vi "GetState.vi"(6 "error in (no error)":errorcluster, 8 "IMU Channel":tag="A/I2C", 9 "LIDAR Channel":tag="B/I2C") -> (0 "error out":errorcluster, 1 "Height":dbl, 2 "Angular Velocity":dbl[](array[numeric]), 3 "Acceleration":dbl[](array[numeric]))   [LabVIEW 2017]
panel:
  in  "Acceleration Factor (experimentally determined)":dbl format="%#_13g"
  out "MyRIO Acceleration":dbl[](array[numeric])
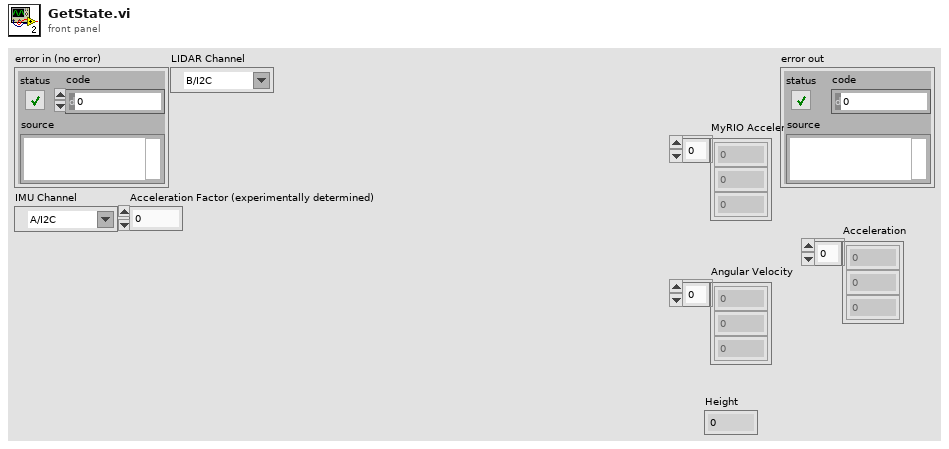
[diagram p1: front panel]
types:
  T1 = cluster{"X-axis":i16, "Y-axis":i16, "Z-axis":i16}
  T2 = cluster{"X-Axis":dbl, "Y-Axis":dbl, "Z-Axis":dbl}
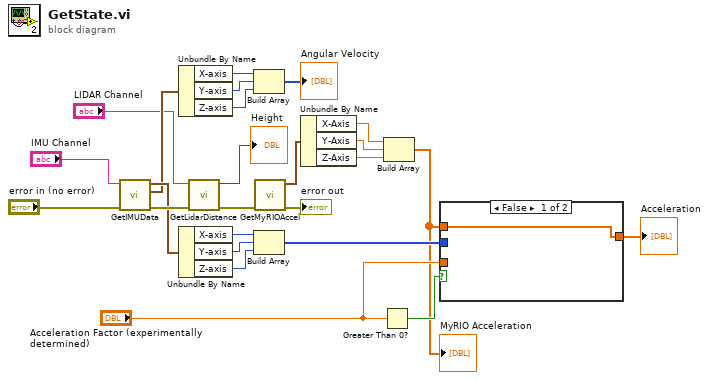
[diagram p0: block diagram]
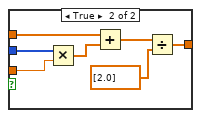
[diagram p2: hidden frame]
diagram:
  n1 = call "GetIMUData.vi"("error in (no error)"="error in (no error)", "Channel Name"="IMU Channel") -> ("error out"=w23:errorcluster, "GyroData"=w18:T1, "AccelData"=w19:T1)  [unwired: 7 in]
  n2 = Unbundle By Name(w18) -> ("X-axis"=w12:i16, "Y-axis"=w11:i16, "Z-axis"=w10:i16)
  n3 = Unbundle By Name(w19) -> ("X-axis"=w8:i16, "Y-axis"=w7:i16, "Z-axis"=w6:i16)
  n4 = call "GetLidarDistance.vi"("error in"=w23, "Channel Name"="LIDAR Channel") -> ("error out"=w22:errorcluster, "(hi.lo)"=→"Height":u16)  [unwired: 8 in]
  n5 = Build Array(w12, w11, w10) -> (→"Angular Velocity":i16[])
  n6 = Build Array(w8, w7, w6) -> (w3:i16[])
  n7 = call "GetMyRIOAccel.vi"("error in (no error)"=w22) -> ("error out"=→"error out":errorcluster, "output cluster"=w20:T2)  [unwired: 9 in]
  n8 = Unbundle By Name(w20) -> ("X-Axis"=w15:dbl, "Y-Axis"=w14:dbl, "Z-Axis"=w13:dbl)
  n9 = Greater Than 0?(x="Acceleration Factor (experimentally determined)") -> (x > 0?=w5:bool)
  n10 = Build Array(w15, w14, w13) -> (w2:dbl[])
  "MyRIO Acceleration" <- w2
  n11 = case shown="False" w5 {
    tunnel: "Acceleration Factor (experimentally determined)" -> [_ w33]
    tunnel: w3 -> [_ w32]
    tunnel: w2 -> [w26 w30]
    tunnel: [w26 w27] -> w1
    frame False {
    }
    frame True {
      n12 = Multiply(x=w32, y=w33) -> (x*y=w31:dbl[])
      n13 = Add(x=w30, y=w31) -> (x+y=w29:dbl[])
      n14 = Divide(x=w29, y=dbl[] [2.0]) -> (x/y=w27:dbl[])
    }
  }
  "Acceleration" <- w1
